vi "Button_combination.vi"(1 "Right 2":bool, 2 "Right 1":bool, 3 "Left 2":bool, 4 "Left 1":bool) -> (0 "Combination":bool)   [LabVIEW 2013]
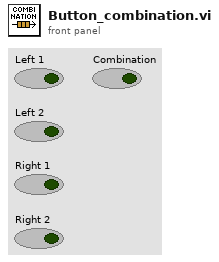
[diagram p1: front panel]
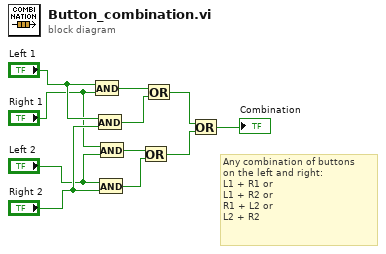
[diagram p0: block diagram]
diagram:
  # "Any combination of buttons \non the left and right:\nL1 + R1 or\nL1 + R2 or\nR1 + L2 or\nL2 + R2"
  n1 = And(x="Left 1", y="Right 1") -> (x .and. y?=w7:bool)
  n2 = And(x="Left 1", y="Right 2") -> (x .and. y?=w6:bool)
  n3 = And(x="Left 2", y="Right 2") -> (x .and. y?=w4:bool)
  n4 = And(x="Right 1", y="Left 2") -> (x .and. y?=w5:bool)
  n5 = Or(x=w5, y=w4) -> (x .or. y?=w2:bool)
  n6 = Or(x=w7, y=w6) -> (x .or. y?=w3:bool)
  n7 = Or(x=w3, y=w2) -> (x .or. y?=→"Combination":bool)
